vi "Send Software Trigger.vi"(8 "error in (no error)":errorcluster, 11 "VISA resource name":refnum<visa-resource-name>) -> (0 "error out":errorcluster, 3 "VISA resource name out":refnum<visa-resource-name>)   [LabVIEW 2017, in "ADCMT 6240.lvlib"]
doc: "This VI sends a software bus trigger to the instrument. \nIt doesn't depend on the trigger mode is auto or manual, the software bus trigger is used for starting sweep. \nAdditionally you can use software bus triggers to trigger multipoint measurements. You must first set Trigger Mode to Manual in the <B>Configure Trigger VI</B>, and specify the Sample Count in the <B>Configure Multipoint VI</B>. After the call to <B>Enable Output VI</B>, send the software bus triggers by calling this VI repeatedly. When triggers are complete, call the <B>Fetch Measurement VI</B> in a loop until completion."
uses:
  ADCMT 6240.lvlib
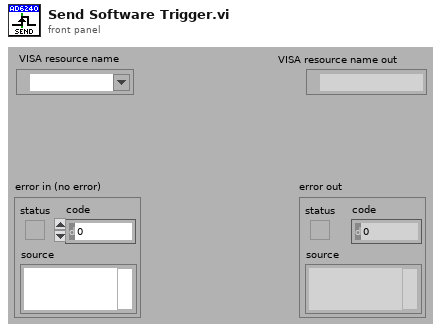
[diagram p1: front panel]
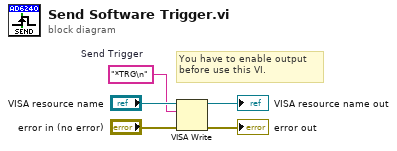
[diagram p0: block diagram]
diagram:
  w3 = "*TRG\n"  # Send Trigger
  # "You have to enable output \nbefore use this VI."
  n1 = VISA Write(VISA resource name="VISA resource name", write buffer=w3, error in (no error)="error in (no error)") -> (VISA resource name out=→"VISA resource name out":refnum<visa-resource-name>, error out=→"error out":errorcluster)  [unwired: 1 out]
